vi "Write Read.vi"(8 "error in (no error)":errorcluster, 10 "write string":string, 11 "VISA Refnum in":refnum<visa-resource-name>) -> (0 "error out":errorcluster, 2 "read string":string, 3 "VISA Refnum out":refnum<visa-resource-name>)   [LabVIEW 2018, in "Huber Unistat 410 TCU.lvlib"]
uses:
  Huber Unistat 410 TCU.lvlib
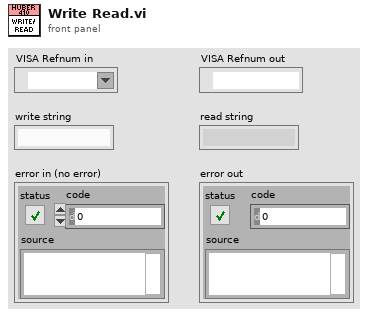
[diagram p1: front panel]
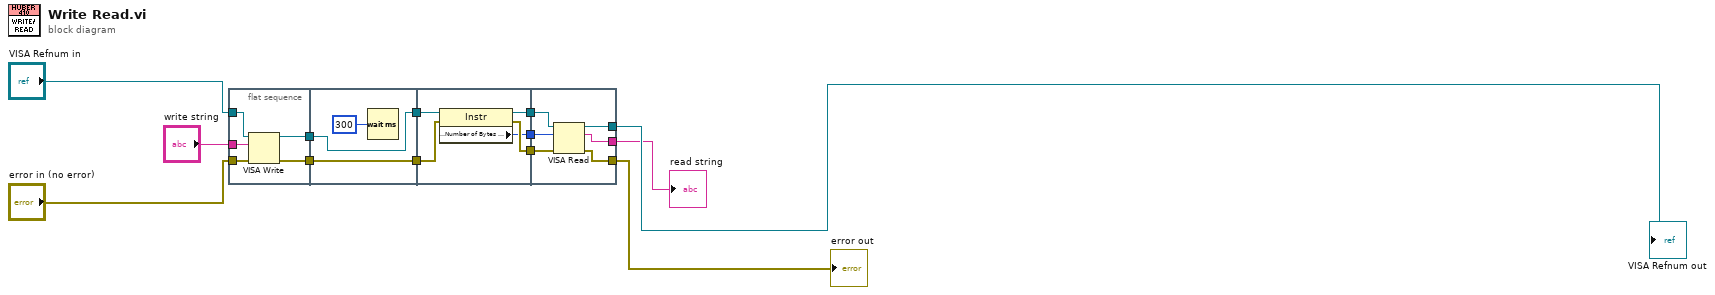
[diagram p0: block diagram]
diagram:
  n1 = flat-sequence {
    tunnel: "write string" -> [w18]
    tunnel: [w17] -> w13
    tunnel: [w16] -> w12
    tunnel: "VISA Refnum in" -> [w15]
    tunnel: "error in (no error)" -> [w14]
    tunnel: w13 -> [w20]
    tunnel: w12 -> [w19]
    tunnel: [w20] -> w11
    tunnel: [w19] -> w10
    tunnel: [w24] -> w9
    tunnel: [w23] -> w8
    tunnel: [w22] -> w7
    tunnel: w11 -> [w26]
    tunnel: w10 -> [w25]
    tunnel: [w32] -> w5
    tunnel: [w31] -> w4
    tunnel: [w30] -> w6
    tunnel: w9 -> [w29]
    tunnel: w8 -> [w28]
    tunnel: w7 -> [w27]
    frame #0 {
      n2 = VISA Write(VISA resource name=w15, write buffer=w18, error in (no error)=w14) -> (VISA resource name out=w17:refnum<visa-resource-name>, error out=w16:errorcluster)  [unwired: 1 out]
    }
    frame #1 {
      n3 = Wait (ms)(milliseconds to wait=u32 300) -> ()  [unwired: 1 out]
    }
    frame #2 {
      n4 = property class="Instr"(reference=w26, error in=w25) -> (reference out=w24:refnum<visa-resource-name>, error out=w23:errorcluster, "Serial Settings:Number of Bytes at Serial Port"=w22:u32)
    }
    frame #3 {
      n5 = VISA Read(VISA resource name=w29, byte count=w27, error in (no error)=w28) -> (VISA resource name out=w30:refnum<visa-resource-name>, read buffer=w31:string, error out=w32:errorcluster)  [unwired: 1 out]
    }
  }
  "VISA Refnum out" <- w6
  "error out" <- w5
  "read string" <- w4
